vi "Verify if the Global Ch Exist.vi"(0 "Global Channels":refnum<k21>, 11 "error in (no error)":errorcluster) -> (15 "error out":errorcluster)   [LabVIEW 2021]
doc: "This VI verifies if the global channel exist in NI MAX and returns error"
uses:
  <vilib>/Utility/error.llb/Error Cluster From Error Code.vi
  <vilib>/ErrorRing/Error Ring.xnode
  <resource>/objmgr/daqmx.rc
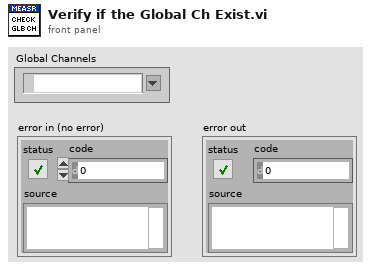
[diagram p1: front panel]
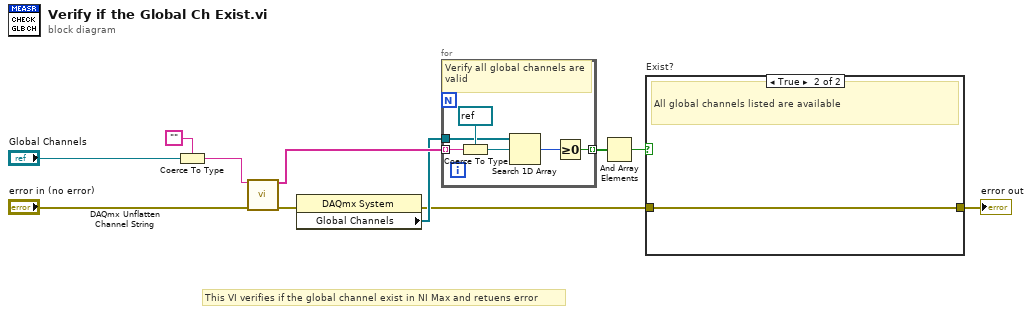
[diagram p0: block diagram]
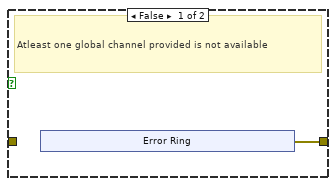
[diagram p2: hidden frame]
diagram:
  # "This VI verifies if the global channel exist in NI Max and retuens error"
  n1 = Coerce To Type(0:"Global Channels", 1:"") -> (2:w6:string)
  n2 = call <vilib>:"DAQmx Unflatten Channel String.vi"("names in"=w6, "error in"="error in (no error)") -> ("names out"=w10:string[], "error out"=w9:errorcluster)  [unwired: 12 in]
  n3 = property class="DAQmx System"(error in=w9) -> (error out=w4:errorcluster, "Global Channels"=w7:refnum<k21>[])  [unwired: 1 in, 1 out]
  n4 = for {
    tunnel: w7 -> [w12]
    tunnel: [w16] -> w11 mode=indexing
    tunnel: w10 -> [w15] mode=indexing
    # "Verify all global channels are valid"
    n5 = Coerce To Type(0:w15, 1:refnum<k21> refnum) -> (2:w14:refnum<k21>)
    n6 = Search 1D Array(1D array=w12, element=w14) -> (index of element=w17:i32)  [unwired: 1 in]
    n7 = Greater Or Equal To 0?(x=w17) -> (x >= 0?=w16:bool)
  }
  n8 = And Array Elements(Boolean array=w11) -> (logical AND=w2:bool)
  n9 = case "Exist?" shown="True" w2 {
    tunnel: w4 -> [_ w23]
    tunnel: [w18 w23] -> w3
    frame False {
      # "Atleast one global channel provided is not available"
      n10 = xnode "Error Ring"() -> ("error out"=w18:errorcluster)
    }
    frame True {
      # "All global channels listed are available"
    }
  }
  "error out" <- w3
